vi "OpenTalonDrive.vi"   [LabVIEW 2016]
uses:
  <vilib>/Rock Robotics/WPI/ThirdParty/CanMotor/TalonSRX/WPI_CANTalonSRX_APIControlMode.ctl
  <vilib>/Rock Robotics/WPI/SafetyOutput/WPI_SafetyOutputConfigMenu.ctl
  <vilib>/Rock Robotics/WPI/ThirdParty/CanMotor/TalonSRX/WPI_CANTalonSRX_APIFeedbackSelect.ctl
types:
  T1 = typedef "WPI_CANTalonSRX_APIFeedbackSelect.ctl" = enum16{"Digital Quadrature Encoder", "Analog Potentiometer", "Analog Encoder", "Count on Quad-A (Rising-Edge)", "Count on Quad-A (Falling-Edge)", "CTR Magnetic Enc (Absolute)", "CTR Magnetic Enc (Relative)", "Pulse Width"}
  T2 = typedef "WPI_SafetyOutputConfigMenu.ctl" = enum16{"Enable", "Disable"}
  T3 = typedef "WPI_CANTalonSRX_APIControlMode.ctl" = enum8{"Percent VBus", "Speed", "Position", "Slave", "Unchanged / Invalid", "Voltage Compensation", "Current", "Motion Profile", "Motion Magic"}
  T4 = typedef "WPI_MotorControlDeviceRef.ctl" = cluster{"DeviceStatus":errorcluster, "Type":T5, "PWM":cluster{"PWM Channel":T6, "DeadBand":T7}, "CAN":cluster{"Device Number":u8, "SetOutput VI Ref":variant, "GetOutput VI Ref":variant, "Enable VI Ref":variant, "Disable VI Ref":variant, "Data":variant}, "Invert":bool}
  T5 = typedef "WPI_MotorControlType.ctl" = enum16{"PWM", "CAN"}
  T6 = typedef "FPGA_DIOPWMChannel.ctl" = enum8{"PWM 0", "PWM 1", "PWM 2", "PWM 3", "PWM 4", "PWM 5", "PWM 6", "PWM 7", "PWM 8", "PWM 9", "PWM MXP 0", "PWM MXP 1", "PWM MXP 2", "PWM MXP 3", "PWM MXP 4", "PWM MXP 5", "PWM MXP 6", "PWM MXP 7", "PWM MXP 8", "PWM MXP 9", "Invalid"}
  T7 = typedef "WPI_PWMDeadband.ctl" = cluster{"Name":string, "maxPositivePwm":i32, "minPositivePwm":i32, "centerPwm":i32, "maxNegativePwm":i32, "minNegativePwm":i32, "angularRange":u16}
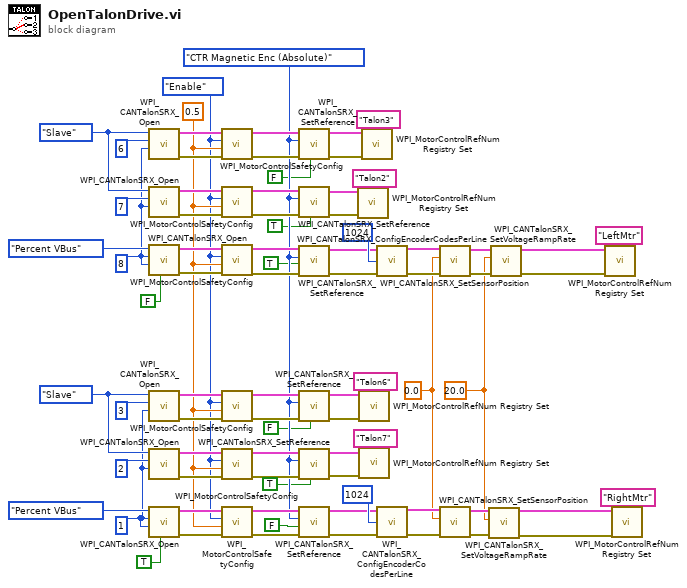
[diagram p0: block diagram]
diagram:
  w13 = 20.0 ("Throttle Ramp Rate (percent/s)")
  w33 = WPI_CANTalonSRX_APIFeedbackSelect."CTR Magnetic Enc (Absolute)" ("Feedback Reference")
  w50 = WPI_SafetyOutputConfigMenu."Enable" ("mode")
  w18 = 0.0 ("New Sensor Position")
  w20 = u8 1 ("Device Number")
  w65 = WPI_CANTalonSRX_APIControlMode."Slave" ("Control Mode")
  w51 = 0.5 ("timeout (s)")
  w19 = u8 8 ("Device Number")
  w79 = WPI_CANTalonSRX_APIControlMode."Slave" ("Control Mode")
  n1 = call <vilib>:"WPI_CANTalonSRX_Open.vi"("Master Device Number"=w19, "Device Number"=u8 6, "Control Mode"=w79) -> ("error out"=w72:errorcluster, "CAN Talon SRX Ref"=w73:T4)  [unwired: 7 in]
  n2 = call <vilib>:"WPI_CANTalonSRX_Open.vi"("Master Device Number"=w19, "Device Number"=u8 7, "Control Mode"=w79) -> ("error out"=w70:errorcluster, "CAN Talon SRX Ref"=w71:T4)  [unwired: 7 in]
  n3 = call <vilib>:"WPI_CANTalonSRX_Open.vi"("Invert"=FALSE, "Master Device Number"=w19, "Device Number"=w19, "Control Mode"=WPI_CANTalonSRX_APIControlMode."Percent VBus") -> ("error out"=w74:errorcluster, "CAN Talon SRX Ref"=w75:T4)  [unwired: 6 in]
  n4 = call <vilib>:"WPI_CANTalonSRX_Open.vi"("Master Device Number"=w20, "Device Number"=u8 3, "Control Mode"=w65) -> ("error out"=w58:errorcluster, "CAN Talon SRX Ref"=w59:T4)  [unwired: 7 in]
  n5 = call <vilib>:"WPI_CANTalonSRX_Open.vi"("Master Device Number"=w20, "Device Number"=u8 2, "Control Mode"=w65) -> ("error out"=w56:errorcluster, "CAN Talon SRX Ref"=w57:T4)  [unwired: 7 in]
  n6 = call <vilib>:"WPI_CANTalonSRX_Open.vi"("Invert"=TRUE, "Master Device Number"=w20, "Device Number"=w20, "Control Mode"=WPI_CANTalonSRX_APIControlMode."Percent VBus") -> ("error out"=w60:errorcluster, "CAN Talon SRX Ref"=w61:T4)  [unwired: 6 in]
  n7 = call <vilib>:"WPI_MotorControlSafetyConfig.vi"("error in (no error)"=w72, "timeout (s)"=w51, "mode"=w50, "MotorControlDevRef"=w73) -> ("error out"=w48:errorcluster, "MotorControlDevRef"=w49:T4)  [unwired: 6 in]
  n8 = call <vilib>:"WPI_MotorControlSafetyConfig.vi"("error in (no error)"=w70, "timeout (s)"=w51, "mode"=w50, "MotorControlDevRef"=w71) -> ("error out"=w46:errorcluster, "MotorControlDevRef"=w47:T4)  [unwired: 6 in]
  n9 = call <vilib>:"WPI_MotorControlSafetyConfig.vi"("error in (no error)"=w74, "timeout (s)"=w51, "mode"=w50, "MotorControlDevRef"=w75) -> ("error out"=w36:errorcluster, "MotorControlDevRef"=w37:T4)  [unwired: 6 in]
  n10 = call <vilib>:"WPI_MotorControlSafetyConfig.vi"("error in (no error)"=w58, "timeout (s)"=w51, "mode"=w50, "MotorControlDevRef"=w59) -> ("error out"=w43:errorcluster, "MotorControlDevRef"=w42:T4)  [unwired: 6 in]
  n11 = call <vilib>:"WPI_MotorControlSafetyConfig.vi"("error in (no error)"=w56, "timeout (s)"=w51, "mode"=w50, "MotorControlDevRef"=w57) -> ("error out"=w45:errorcluster, "MotorControlDevRef"=w44:T4)  [unwired: 6 in]
  n12 = call <vilib>:"WPI_MotorControlSafetyConfig.vi"("error in (no error)"=w60, "timeout (s)"=w51, "mode"=w50, "MotorControlDevRef"=w61) -> ("error out"=w40:errorcluster, "MotorControlDevRef"=w41:T4)  [unwired: 6 in]
  n13 = call <vilib>:"WPI_CANTalonSRX_SetReference.vi"("Reverse Closed-Loop Output"=FALSE, "error in (no error)"=w48, "Feedback Reference"=w33, "CAN Talon SRX Ref"=w49) -> ("error out"=w25:errorcluster, "CAN Talon SRX Ref"=w24:T4)  [unwired: 6 in]
  n14 = call <vilib>:"WPI_CANTalonSRX_SetReference.vi"("Reverse Closed-Loop Output"=TRUE, "error in (no error)"=w46, "Feedback Reference"=w33, "CAN Talon SRX Ref"=w47) -> ("error out"=w27:errorcluster, "CAN Talon SRX Ref"=w26:T4)  [unwired: 6 in]
  n15 = call <vilib>:"WPI_CANTalonSRX_SetReference.vi"("error in (no error)"=w36, "Reverse Feedback Sensor"=TRUE, "Feedback Reference"=w33, "CAN Talon SRX Ref"=w37) -> ("error out"=w34:errorcluster, "CAN Talon SRX Ref"=w35:T4)  [unwired: 6 in]
  n16 = call <vilib>:"WPI_CANTalonSRX_SetReference.vi"("Reverse Closed-Loop Output"=FALSE, "error in (no error)"=w43, "Feedback Reference"=w33, "CAN Talon SRX Ref"=w42) -> ("error out"=w29:errorcluster, "CAN Talon SRX Ref"=w28:T4)  [unwired: 6 in]
  n17 = call <vilib>:"WPI_CANTalonSRX_SetReference.vi"("Reverse Closed-Loop Output"=TRUE, "error in (no error)"=w45, "Feedback Reference"=w33, "CAN Talon SRX Ref"=w44) -> ("error out"=w32:errorcluster, "CAN Talon SRX Ref"=w31:T4)  [unwired: 6 in]
  n18 = call <vilib>:"WPI_CANTalonSRX_SetReference.vi"("error in (no error)"=w40, "Reverse Feedback Sensor"=FALSE, "Feedback Reference"=w33, "CAN Talon SRX Ref"=w41) -> ("error out"=w38:errorcluster, "CAN Talon SRX Ref"=w39:T4)  [unwired: 6 in]
  n19 = call <vilib>:"WPI_MotorControlRefNum Registry Set.vi"("error in (no error)"=w27, "refnum name"="Talon2", "MotorControlDevRef"=w26) -> ()  [unwired: 7 in, 2 out]
  n20 = call <vilib>:"WPI_MotorControlRefNum Registry Set.vi"("error in (no error)"=w29, "refnum name"="Talon6", "MotorControlDevRef"=w28) -> ()  [unwired: 7 in, 2 out]
  n21 = call <vilib>:"WPI_MotorControlRefNum Registry Set.vi"("error in (no error)"=w32, "refnum name"="Talon7", "MotorControlDevRef"=w31) -> ()  [unwired: 7 in, 2 out]
  n22 = call <vilib>:"WPI_MotorControlRefNum Registry Set.vi"("error in (no error)"=w25, "refnum name"="Talon3", "MotorControlDevRef"=w24) -> ()  [unwired: 7 in, 2 out]
  n23 = call <vilib>:"WPI_CANTalonSRX_ConfigEncoderCodesPerLine.vi"("CAN Talon SRX Ref"=w35, "Number Encoder Lines\n(Counts Per Rotation)"=u32 1024 ("Number Encoder Lines\n(Counts Per Rotation)"), "error in (no error)"=w34) -> ("CAN Talon SRX Ref"=w67:T4, "error out"=w68:errorcluster)  [unwired: 11 in]
  n24 = call <vilib>:"WPI_CANTalonSRX_ConfigEncoderCodesPerLine.vi"("CAN Talon SRX Ref"=w39, "Number Encoder Lines\n(Counts Per Rotation)"=u32 1024 ("Number Encoder Lines\n(Counts Per Rotation)"), "error in (no error)"=w38) -> ("CAN Talon SRX Ref"=w53:T4, "error out"=w54:errorcluster)  [unwired: 11 in]
  n25 = call <vilib>:"WPI_CANTalonSRX_SetSensorPosition.vi"("error in (no error)"=w68, "New Sensor Position"=w18, "CAN Talon SRX Ref"=w67) -> ("error out"=w14:errorcluster, "CAN Talon SRX Ref"=w15:T4)  [unwired: 7 in]
  n26 = call <vilib>:"WPI_CANTalonSRX_SetSensorPosition.vi"("error in (no error)"=w54, "New Sensor Position"=w18, "CAN Talon SRX Ref"=w53) -> ("error out"=w17:errorcluster, "CAN Talon SRX Ref"=w16:T4)  [unwired: 7 in]
  n27 = call <vilib>:"WPI_CANTalonSRX_SetVoltageRampRate.vi"("error in (no error)"=w17, "Throttle Ramp Rate (percent/s)"=w13, "CAN Talon SRX Ref"=w16) -> ("error out"=w9:errorcluster, "CAN Talon SRX Ref"=w10:T4)  [unwired: 7 in]
  n28 = call <vilib>:"WPI_CANTalonSRX_SetVoltageRampRate.vi"("error in (no error)"=w14, "Throttle Ramp Rate (percent/s)"=w13, "CAN Talon SRX Ref"=w15) -> ("error out"=w12:errorcluster, "CAN Talon SRX Ref"=w11:T4)  [unwired: 7 in]
  n29 = call <vilib>:"WPI_MotorControlRefNum Registry Set.vi"("error in (no error)"=w12, "refnum name"="LeftMtr" ("Ref Name 1"), "MotorControlDevRef"=w11) -> ()  [unwired: 7 in, 2 out]
  n30 = call <vilib>:"WPI_MotorControlRefNum Registry Set.vi"("error in (no error)"=w9, "refnum name"="RightMtr" ("Ref Name 2"), "MotorControlDevRef"=w10) -> ()  [unwired: 7 in, 2 out]
